vi "Digital Read Port.vi"(0 "Arduino Resource":T1={"VISA resource"="", "Board Type"=enum."Uno", "Connection Type"=enum."USB / Serial", "Bytes Per Packet (15)"=15}, 11 "error in":errorcluster) -> (4 "Arduino Resource":T1={"VISA resource"="", "Board Type"=enum."Uno", "Connection Type"=enum."USB / Serial", "Bytes Per Packet (15)"=15}, 8 "Digital Port":bool[](array[boolean]), 15 "error out":errorcluster)   [LabVIEW 2011, in "LabVIEW Interface for Arduino.lvlib"]
doc: "Reads the digital value of the selected Arduino digital input pin (D0 - D13). The pin must fist be configured as an input using the Arduino Set Digital Pin Mode VI."
uses:
  <vilib>/LabVIEW Interface for Arduino/LabVIEW Interface for Arduino.lvlib
  <vilib>/LabVIEW Interface for Arduino/Private/Type Defs/Arduino Resource.ctl
  <vilib>/LabVIEW Interface for Arduino/Private/Type Defs/Board Type.ctl
  <vilib>/LabVIEW Interface for Arduino/Private/Type Defs/Command.ctl
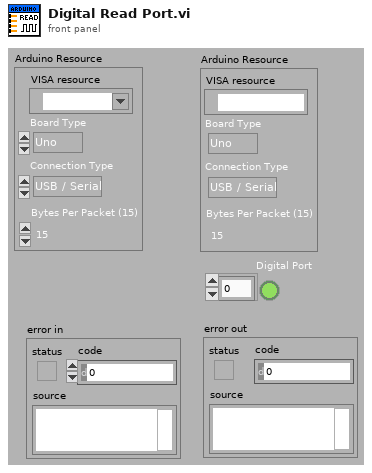
[diagram p1: front panel]
types:
  T1 = typedef "LabVIEW Interface for Arduino.lvlib/Arduino Resource.ctl" = cluster{"VISA resource":refnum<visa-resource-name>, "Board Type":T2, "Connection Type":enum8{"USB / Serial"}, "Bytes Per Packet (15)":u8}
  T2 = typedef "LabVIEW Interface for Arduino.lvlib/Board Type.ctl" = enum16{"Uno", "Dimuelanove w/Atmega 328", "Mega 2560"}
  T3 = typedef "LabVIEW Interface for Arduino.lvlib/Command.ctl" = enum8{"setArduinoMode", "flushSerial", "setPinMode", "digitalWritePin", "digitalWritePort", "tone", "digitalReadPin", "digitalReadPort", "analogReadPin", "analogReadPort", "pwmWritePin", "pwmWritePort", "sevenSegment_Configure", "sevenSegment_Write", "I2C Init", "I2C Write", "I2C Read", "SPI Init", "SPI Set Bit Order", "SPI Set Clock Divider", "SPI Set Data Mode", "SPI Send / Receive", "SPI Close", "Servo Set Num Servos", "Servo Config Servo", "Servo Write Angle", "Servo Read Angle", "Servo Write Pulse Width", "Servo Read Pulse Width", "Servo Detach", "LCD Init", "LCD Set Size", "LCD Set Cursor Mode", "LCD Clear", "LCD Set Cursor Position", "LCD Print", "LCD Display Power", "LCD Scroll Display", "LCD Autoscroll", "LCD Print Direction", "LCD Create Custom Char", "LCD Print Custom Char", "contAcqOn", "contAcqOff", "getFirmwareVersion", "FiniteSampleStart"}
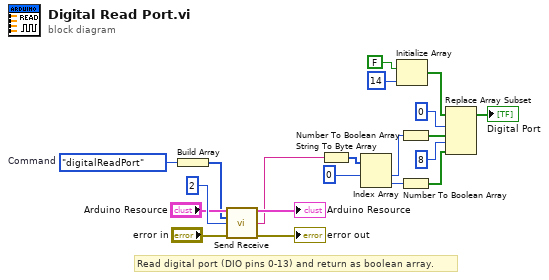
[diagram p0: block diagram]
diagram:
  w19 = Command."digitalReadPort"  # Command
  # "Read digital port (DIO pins 0-13) and return as boolean array."
  n1 = Build Array(w19) -> (w13:T3[])
  n2 = call <vilib>:"Send Receive.vi"("Arduino Resource"="Arduino Resource", "Data"=w13, "Bytes To Read (0)"=u32 2, "error in"="error in") -> ("Arduino Resource"=→"Arduino Resource":T1, "Read Buffer"=w12:string, "error out"=→"error out":errorcluster)  [unwired: 9 in]
  n3 = String To Byte Array(string=w12) -> (unsigned byte array=w20:u8[])
  n4 = Index Array(array=w20, index #1=0 ("index")) -> (element #1=w11:u8, element #2=w10:u8)  [unwired: 1 in]
  n5 = Initialize Array(FALSE, 14 ("dimension size")) -> (w8:bool[])
  n6 = Number To Boolean Array(number=w11) -> (Boolean array=w5:bool[])
  n7 = Number To Boolean Array(number=w10) -> (Boolean array=w2:bool[])
  n8 = Replace Array Subset(array=w8, new element #1=w5, index #1=0 ("index"), new element #2=w2, index #2=8 ("index")) -> (→"Digital Port":bool[])
